vi "Do.vi"(8 "error in (no error)":errorcluster, 10 "Actor in":refnum<class "Actor.lvclass">, 11 "Class Loading Progress Msg in":refnum<class "Class Loading Progress Msg.lvclass">) -> (0 "error out":errorcluster, 2 "Actor out":refnum<class "Actor.lvclass">)   [LabVIEW 2023, in "Class Loader.lvlib" / "Class Loading Progress Msg.lvclass"]
doc: "This VI delivers the message to the actor by calling the appropriate method(s) on the actor."
uses:
  Class Loading Progress Msg.lvclass
  <vilib>/ActorFramework/Actor/Actor.lvclass
  Class Loading Progress Msg.lvclass/Class Loading Progress Msg.ctl
  Class Loader Interfaces/Class Loader Interfaces.lvclass
  5939451c-e789-4642-81e2-21d1869227c8.vi
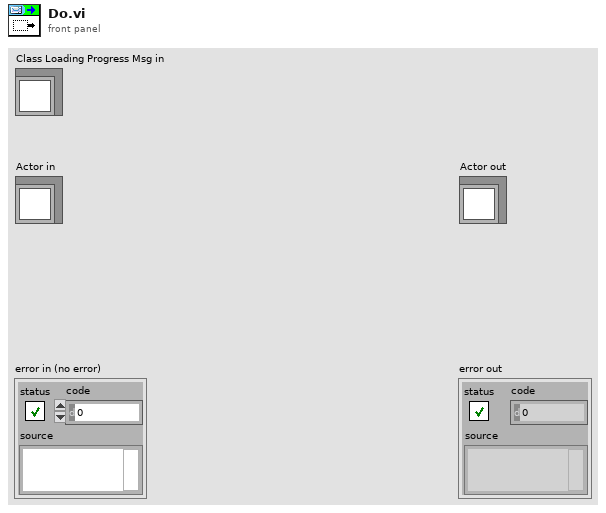
[diagram p1: front panel]
types:
  T1 = typedef "Class Loader.lvlib/Class Loader.lvclass/Loading Progress.ctl" = dbl
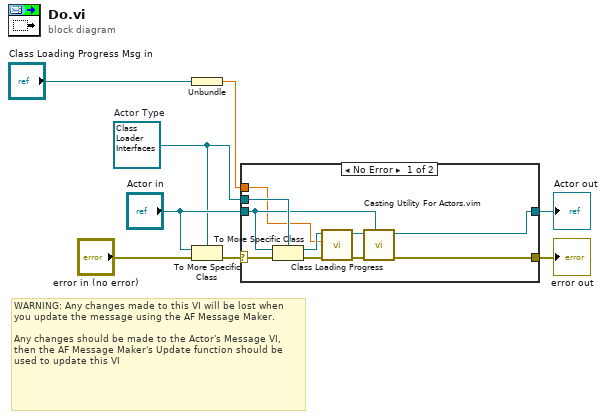
[diagram p0: block diagram]
diagram:
  w3 = refnum<class "Class Loader Interfaces.lvclass"> refnum  # Actor Type
  # "WARNING: Any changes made to this VI will be lost when you update the message using the AF Message Maker.\n\nAny changes should be made to the Actor's Message VI, then the AF Message Maker's Update function should be used to update this VI"
  n1 = Unbundle("Class Loading Progress Msg in") -> (w2:T1)
  n2 = To More Specific Class(target class=w3, reference="Actor in", error in="error in (no error)") -> (error out=w7:errorcluster)  [unwired: 1 out]
  n3 = case shown="No Error" w7 {
    selector: w7 -> [w14 w20]
    tunnel: [w16 w20] -> w6
    tunnel: [w15 w19] -> w5
    tunnel: "Actor in" -> [w17 w19]
    tunnel: w3 -> [w18 _]
    tunnel: w2 -> [w9 _]
    frame No Error {
      n4 = To More Specific Class ("Actor Cast")(target class=w18, reference=w17, error in=w14) -> (specific class reference=w13:refnum<class "Class Loader Interfaces.lvclass">, error out=w12:errorcluster)
      n5 = call-dynamic "Class Loading Progress.vi"("error in (no error)"=w12, "Progress (%)"=w9, "Class Loader Interfaces in"=w13) -> ("error out"=w10:errorcluster, "Class Loader Interfaces out"=w11:refnum<class "Class Loader Interfaces.lvclass">)  [unwired: 7 in]
      n6 = call "Casting Utility For Actors.vim"("type"=w17, "error in (no error)"=w10, "Actor in"=w11) -> ("error out"=w16:errorcluster, "Actor out"=w15:refnum<class "Actor.lvclass">)  [unwired: 7 in]
    }
    frame Error {
    }
  }
  "error out" <- w6
  "Actor out" <- w5
